vi "HFRR ADV v025 new software.vi"() -> ()   [LabVIEW 2025] (continued)
              n1908 = local write "Numeric 12"(w2274) -> ()
              n1909 = String Length(string=w2275) -> (length=w2277:i32)
              n1910 = Greater?(x=w2277, y=1) -> (0:w2273:bool)
            }
            n1911 = while {
              tunnel: w2248 -> [w2284]
              i -> [w2280]
              stop <- w2279 continue-if-true
              (unwired) TRUE ("line mode (F)")
              n1912 = Read from Text File "Read File"(file (use dialog)=w2284) -> (text=w2281:string)  [unwired: 3 in, 3 out]
              n1913 = local write "Numeric 13"(w2280) -> ()
              n1914 = String Length(string=w2281) -> (length=w2283:i32)
              n1915 = Greater?(x=w2283, y=1) -> (0:w2279:bool)
            }
            n1916 = String To Path(string=w2247) -> (path=w2255:path)
            n1917 = Open/Create/Replace File "Open File"(file path (use dialog)=w2255) -> (refnum out=w2251:refnum<file>)  [unwired: 5 in, 2 out]
            n1918 = while {
              tunnel: w2251 -> [w2266]
              i -> [w2262]
              stop <- w2261 continue-if-true
              (unwired) TRUE ("line mode (F)")
              n1919 = Read from Text File "Read File"(file (use dialog)=w2266) -> (text=w2263:string)  [unwired: 3 in, 3 out]
              n1920 = local write "Numeric 8"(w2262) -> ()
              n1921 = String Length(string=w2263) -> (length=w2265:i32)
              n1922 = Greater?(x=w2265, y=1) -> (0:w2261:bool)
            }
          }
          frame #1 {
            w2436 = FALSE ("ACTUAL   MERGE")
            # "Sample Temp"
            # "ECR"
            # "COF"
            # "Time\nCOF\nFF\nTemp"
            n1923 = case shown="True" w2309 {
              tunnel: [w2456 w2457] -> w2310
              frame False {
                n1924 = local read "string1"() -> (w2456:string)
              }
              frame True {
                n1925 = local read "String Indicator 4"() -> (w2457:string)
              }
            }
            n1926 = local read "string1 3"() -> (w2354:string)
            n1927 = String To Path(string=w2310) -> (path=w2441:path)
            n1928 = String To Path(string=w2354) -> (path=w2452:path)
            n1929 = local read "Numeric 12"() -> (w2438:i32)
            n1930 = local read "Numeric 8"() -> (w2440:i32)
            n1931 = local read "string1 2"() -> (w2355:string)
            n1932 = local read "string1 4"() -> (w2353:string)
            n1933 = Open/Create/Replace File "Open File"(file path (use dialog)=w2441) -> (refnum out=w2455:refnum<file>, error out=w2454:errorcluster)  [unwired: 5 in, 1 out]
            n1934 = Open/Create/Replace File "Open File"(file path (use dialog)=w2452) -> (refnum out=w2448:refnum<file>, error out=w2449:errorcluster)  [unwired: 5 in, 1 out]
            n1935 = for {
              N: w2440 -> [_]
              tunnel: w2455 -> [w2603]
              tunnel: w2454 -> [w2602]
              tunnel: [w2592] -> w2367 mode=indexing
              tunnel: [w2590] -> w2424 mode=indexing
              tunnel: [w2591] -> w2419 mode=indexing
              tunnel: w2436 -> [_]
              tunnel: [w2584] -> w2421 mode=indexing
              tunnel: [w2580] -> w2390 mode=indexing
              tunnel: [w2576] -> w2365 mode=indexing
              tunnel: [w2572] -> w2346 mode=indexing
              tunnel: [w2567] -> w2306 mode=indexing
              (unwired) TRUE ("line mode (F)")
              # "freq"
              # "Stroke"
              # "Time"
              # "CoF"
              # "Humidity"
              # "Temp"
              # "Air Temp"
              # "ECR"
              n1936 = Read from Text File "Read File"(file (use dialog)=w2603, error in=w2602) -> (text=w2568:string)  [unwired: 2 in, 3 out]
              n1937 = local write "String 6"(w2568) -> ()
              n1938 = String Subset(string=w2568, offset (0)=0, length (rest)=14 ("length (rest)")) -> (substring=w2596:string)
              n1939 = String Subset(string=w2568, offset (0)=35, length (rest)=9 ("length (rest)")) -> (substring=w2593:string)
              n1940 = String Subset(string=w2568, offset (0)=15, length (rest)=9 ("length (rest)")) -> (substring=w2599:string)
              n1941 = Fract/Exp String To Number(string=w2596) -> (number=w2592:dbl)  [unwired: 3 in, 1 out]
              n1942 = Fract/Exp String To Number(string=w2593) -> (number=w2591:dbl)  [unwired: 3 in, 1 out]
              n1943 = Fract/Exp String To Number(string=w2599) -> (number=w2590:dbl)  [unwired: 3 in, 1 out]
              n1944 = String Subset(string=w2568, offset (0)=85, length (rest)=9 ("length (rest)")) -> (substring=w2569:string)
              n1945 = String Subset(string=w2568, offset (0)=25, length (rest)=9 ("length (rest)")) -> (substring=w2575:string)
              n1946 = String Subset(string=w2568, offset (0)=55, length (rest)=9 ("length (rest)")) -> (substring=w2577:string)
              n1947 = String Subset(string=w2568, offset (0)=45, length (rest)=9 ("length (rest)")) -> (substring=w2583:string)
              n1948 = String Subset(string=w2568, offset (0)=65, length (rest)=9 ("length (rest)")) -> (substring=w2589:string)
              n1949 = Fract/Exp String To Number(string=w2575) -> (number=w2572:dbl)  [unwired: 3 in, 1 out]
              n1950 = Fract/Exp String To Number(string=w2569) -> (number=w2567:dbl)  [unwired: 3 in, 1 out]
              n1951 = Fract/Exp String To Number(string=w2577) -> (number=w2576:dbl)  [unwired: 3 in, 1 out]
              n1952 = Fract/Exp String To Number(string=w2583) -> (number=w2580:dbl)  [unwired: 3 in, 1 out]
              n1953 = Fract/Exp String To Number(string=w2589) -> (number=w2586:dbl)  [unwired: 3 in, 1 out]
              n1954 = Add(x=w2586, y=0.0) -> (x+y=w2584:dbl)
            }
            n1955 = for {
              N: w2438 -> [_]
              tunnel: w2449 -> [w2529]
              tunnel: w2448 -> [w2528]
              tunnel: [w2518] -> w2407 mode=indexing
              tunnel: [w2516] -> w2405 mode=indexing
              tunnel: [w2517] -> w2401 mode=indexing
              tunnel: w2436 -> [_]
              tunnel: [w2510] -> w2403 mode=indexing
              tunnel: [w2506] -> w2385 mode=indexing
              tunnel: [w2502] -> w2361 mode=indexing
              tunnel: [w2499] -> w2342 mode=indexing
              tunnel: [w2495] -> w2301 mode=indexing
              (unwired) 9 ("length (rest)")
              (unwired) 9 ("length (rest)")
              (unwired) TRUE ("line mode (F)")
              n1956 = Read from Text File "Read File"(file (use dialog)=w2528, error in=w2529) -> (text=w2496:string)  [unwired: 2 in, 3 out]
              n1957 = local write "String 8"(w2496) -> ()
              n1958 = String Subset(string=w2496, offset (0)=85) -> (substring=w2498:string)  [unwired: 1 in]
              n1959 = String Subset(string=w2496, offset (0)=35, length (rest)=9 ("length (rest)")) -> (substring=w2519:string)
              n1960 = String Subset(string=w2496, offset (0)=55, length (rest)=9 ("length (rest)")) -> (substring=w2504:string)
              n1961 = String Subset(string=w2496, offset (0)=25) -> (substring=w2500:string)  [unwired: 1 in]
              n1962 = String Subset(string=w2496, offset (0)=15, length (rest)=9 ("length (rest)")) -> (substring=w2525:string)
              n1963 = String Subset(string=w2496, offset (0)=0, length (rest)=14 ("length (rest)")) -> (substring=w2522:string)
              n1964 = String Subset(string=w2496, offset (0)=45, length (rest)=9 ("length (rest)")) -> (substring=w2509:string)
              n1965 = String Subset(string=w2496, offset (0)=65, length (rest)=9 ("length (rest)")) -> (substring=w2515:string)
              n1966 = Fract/Exp String To Number(string=w2498) -> (number=w2495:dbl)  [unwired: 3 in, 1 out]
              n1967 = Fract/Exp String To Number(string=w2519) -> (number=w2517:dbl)  [unwired: 3 in, 1 out]
              n1968 = Fract/Exp String To Number(string=w2504) -> (number=w2502:dbl)  [unwired: 3 in, 1 out]
              n1969 = Fract/Exp String To Number(string=w2500) -> (number=w2499:dbl)  [unwired: 3 in, 1 out]
              n1970 = Fract/Exp String To Number(string=w2525) -> (number=w2516:dbl)  [unwired: 3 in, 1 out]
              n1971 = Fract/Exp String To Number(string=w2522) -> (number=w2518:dbl)  [unwired: 3 in, 1 out]
              n1972 = Fract/Exp String To Number(string=w2509) -> (number=w2506:dbl)  [unwired: 3 in, 1 out]
              n1973 = Fract/Exp String To Number(string=w2515) -> (number=w2512:dbl)  [unwired: 3 in, 1 out]
              n1974 = Add(x=w2512, y=0.0) -> (x+y=w2510:dbl)
            }
            n1975 = String To Path(string=w2355) -> (path=w2453:path)
            n1976 = String To Path(string=w2353) -> (path=w2447:path)
            n1977 = local read "Numeric 11"() -> (w2437:i32)
            n1978 = local read "Numeric 13"() -> (w2439:i32)
            n1979 = Open/Create/Replace File "Open File"(file path (use dialog)=w2453) -> (refnum out=w2451:refnum<file>, error out=w2450:errorcluster)  [unwired: 5 in, 1 out]
            n1980 = Open/Create/Replace File "Open File"(file path (use dialog)=w2447) -> (refnum out=w2446:refnum<file>, error out=w2445:errorcluster)  [unwired: 5 in, 1 out]
            n1981 = for {
              N: w2437 -> [_]
              tunnel: w2451 -> [w2566]
              tunnel: w2450 -> [w2565]
              tunnel: [w2555] -> w2417 mode=indexing
              tunnel: [w2553] -> w2415 mode=indexing
              tunnel: [w2554] -> w2410 mode=indexing
              tunnel: w2436 -> [_]
              tunnel: [w2547] -> w2412 mode=indexing
              tunnel: [w2543] -> w2388 mode=indexing
              tunnel: [w2539] -> w2363 mode=indexing
              tunnel: [w2535] -> w2344 mode=indexing
              tunnel: [w2530] -> w2302 mode=indexing
              (unwired) TRUE ("line mode (F)")
              n1982 = Read from Text File "Read File"(file (use dialog)=w2566, error in=w2565) -> (text=w2531:string)  [unwired: 2 in, 3 out]
              n1983 = local write "String 7"(w2531) -> ()
              n1984 = String Subset(string=w2531, offset (0)=85, length (rest)=9 ("length (rest)")) -> (substring=w2534:string)
              n1985 = String Subset(string=w2531, offset (0)=35, length (rest)=9 ("length (rest)")) -> (substring=w2556:string)
              n1986 = String Subset(string=w2531, offset (0)=55, length (rest)=9 ("length (rest)")) -> (substring=w2542:string)
              n1987 = String Subset(string=w2531, offset (0)=25, length (rest)=9 ("length (rest)")) -> (substring=w2536:string)
              n1988 = String Subset(string=w2531, offset (0)=45, length (rest)=9 ("length (rest)")) -> (substring=w2544:string)
              n1989 = String Subset(string=w2531, offset (0)=0, length (rest)=14 ("length (rest)")) -> (substring=w2559:string)
              n1990 = String Subset(string=w2531, offset (0)=15, length (rest)=9 ("length (rest)")) -> (substring=w2562:string)
              n1991 = String Subset(string=w2531, offset (0)=65, length (rest)=9 ("length (rest)")) -> (substring=w2548:string)
              n1992 = Fract/Exp String To Number(string=w2534) -> (number=w2530:dbl)  [unwired: 3 in, 1 out]
              n1993 = Fract/Exp String To Number(string=w2556) -> (number=w2554:dbl)  [unwired: 3 in, 1 out]
              n1994 = Fract/Exp String To Number(string=w2542) -> (number=w2539:dbl)  [unwired: 3 in, 1 out]
              n1995 = Fract/Exp String To Number(string=w2536) -> (number=w2535:dbl)  [unwired: 3 in, 1 out]
              n1996 = Fract/Exp String To Number(string=w2544) -> (number=w2543:dbl)  [unwired: 3 in, 1 out]
              n1997 = Fract/Exp String To Number(string=w2559) -> (number=w2555:dbl)  [unwired: 3 in, 1 out]
              n1998 = Fract/Exp String To Number(string=w2562) -> (number=w2553:dbl)  [unwired: 3 in, 1 out]
              n1999 = Fract/Exp String To Number(string=w2548) -> (number=w2551:dbl)  [unwired: 3 in, 1 out]
              n2000 = Add(x=w2551, y=0.0) -> (x+y=w2547:dbl)
            }
            n2001 = for {
              N: w2439 -> [_]
              tunnel: w2446 -> [w2494]
              tunnel: w2445 -> [w2493]
              tunnel: [w2483] -> w2399 mode=indexing
              tunnel: [w2482] -> w2392 mode=indexing
              tunnel: w2436 -> [_]
              tunnel: [w2471] -> w2397 mode=indexing
              tunnel: [w2476] -> w2394 mode=indexing
              tunnel: [w2472] -> w2384 mode=indexing
              tunnel: [w2467] -> w2359 mode=indexing
              tunnel: [w2463] -> w2340 mode=indexing
              tunnel: [w2458] -> w2300 mode=indexing
              (unwired) 1.0 ("x")
              (unwired) TRUE ("line mode (F)")
              n2002 = Read from Text File "Read File"(file (use dialog)=w2494, error in=w2493) -> (text=w2459:string)  [unwired: 2 in, 3 out]
              n2003 = local write "String 12"(w2459) -> ()
              n2004 = String Subset(string=w2459, offset (0)=85, length (rest)=9 ("length (rest)")) -> (substring=w2461:string)
              n2005 = String Subset(string=w2459, offset (0)=35, length (rest)=9 ("length (rest)")) -> (substring=w2484:string)
              n2006 = String Subset(string=w2459, offset (0)=55, length (rest)=9 ("length (rest)")) -> (substring=w2469:string)
              n2007 = String Subset(string=w2459, offset (0)=25, length (rest)=9 ("length (rest)")) -> (substring=w2465:string)
              n2008 = String Subset(string=w2459, offset (0)=45, length (rest)=9 ("length (rest)")) -> (substring=w2474:string)
              n2009 = String Subset(string=w2459, offset (0)=15, length (rest)=9 ("length (rest)")) -> (substring=w2490:string)
              n2010 = String Subset(string=w2459, offset (0)=0, length (rest)=14 ("length (rest)")) -> (substring=w2487:string)
              n2011 = String Subset(string=w2459, offset (0)=65, length (rest)=9 ("length (rest)")) -> (substring=w2477:string)
              n2012 = Fract/Exp String To Number(string=w2461) -> (number=w2458:dbl)  [unwired: 3 in, 1 out]
              n2013 = Fract/Exp String To Number(string=w2484) -> (number=w2482:dbl)  [unwired: 3 in, 1 out]
              n2014 = Fract/Exp String To Number(string=w2469) -> (number=w2467:dbl)  [unwired: 3 in, 1 out]
              n2015 = Fract/Exp String To Number(string=w2465) -> (number=w2463:dbl)  [unwired: 3 in, 1 out]
              n2016 = Fract/Exp String To Number(string=w2474) -> (number=w2472:dbl)  [unwired: 3 in, 1 out]
              n2017 = Fract/Exp String To Number(string=w2490) -> (number=w2471:dbl)  [unwired: 3 in, 1 out]
              n2018 = Fract/Exp String To Number(string=w2487) -> (number=w2483:dbl)  [unwired: 3 in, 1 out]
              n2019 = Fract/Exp String To Number(string=w2477) -> (number=w2480:dbl)  [unwired: 3 in, 1 out]
              n2020 = Add(x=w2480, y=0.0) -> (x+y=w2476:dbl)
            }
            n2021 = Delete From Array(array=w2342, index=0) -> (array with subset deleted=w2315:dbl[])  [unwired: 1 in, 1 out]
            n2022 = Delete From Array(array=w2405, index=0) -> (array with subset deleted=w2378:dbl[])  [unwired: 1 in, 1 out]
            n2023 = Delete From Array(array=w2385, index=0) -> (array with subset deleted=w2373:dbl[])  [unwired: 1 in, 1 out]
            n2024 = Delete From Array(array=w2403, index=0) -> (array with subset deleted=w2404:dbl[])  [unwired: 1 in, 1 out]
            n2025 = call-poly <vilib>:"Mean.vi"("X"=w2315) -> ("mean"=→"КОФ2 4":dbl)  [unwired: 1 out]
            n2026 = call-poly <vilib>:"Mean.vi"("X"=w2378) -> ("mean"=→"КОФ3":dbl)  [unwired: 1 out]
            n2027 = call-poly <vilib>:"Mean.vi"("X"=w2373) -> ("mean"=→"CP3":dbl)  [unwired: 1 out]
            n2028 = Delete From Array(array=w2367, index=0) -> (array with subset deleted=w2294:dbl[])  [unwired: 1 in, 1 out]
            n2029 = Delete From Array(array=w2306, index=0) -> (array with subset deleted=w2293:dbl[])  [unwired: 1 in, 1 out]
            n2030 = Delete From Array(array=w2346, index=0) -> (array with subset deleted=w2317:dbl[])  [unwired: 1 in, 1 out]
            n2031 = Delete From Array(array=w2424, index=0) -> (array with subset deleted=w2379:dbl[])  [unwired: 1 in, 1 out]
            n2032 = Delete From Array(array=w2390, index=0) -> (array with subset deleted=w2375:dbl[])  [unwired: 1 in, 1 out]
            "array w/ subset deleted" <- w2375
            n2033 = Delete From Array(array=w2421, index=0) -> (array with subset deleted=w2422:dbl[])  [unwired: 1 in, 1 out]
            n2034 = call-poly <vilib>:"Mean.vi"("X"=w2317) -> ("mean"=→"КОФ2 2":dbl)  [unwired: 1 out]
            n2035 = call-poly <vilib>:"Mean.vi"("X"=w2379) -> ("mean"=→"КОФ1":dbl)  [unwired: 1 out]
            n2036 = Bundle "Bundle"(w2294, w2293) -> (w2299:cluster{dbl[], dbl[]})  [unwired: 1 in]
            n2037 = Bundle "Bundle"(w2294, w2422) -> (w2286:cluster{dbl[], dbl[]})  [unwired: 1 in]
            n2038 = Delete From Array(array=w2301, index=0) -> (array with subset deleted=w2289:dbl[])  [unwired: 1 in, 1 out]
            n2039 = Delete From Array(array=w2302, index=0) -> (array with subset deleted=w2291:dbl[])  [unwired: 1 in, 1 out]
            n2040 = Delete From Array(array=w2412, index=0) -> (array with subset deleted=w2413:dbl[])  [unwired: 1 in, 1 out]
            n2041 = Delete From Array(array=w2300, index=0) -> (array with subset deleted=w2287:dbl[])  [unwired: 1 in, 1 out]
            n2042 = Delete From Array(array=w2394, index=0) -> (array with subset deleted=w2395:dbl[])  [unwired: 1 in, 1 out]
            n2043 = Delete From Array(array=w2419, index=0) -> (array with subset deleted=w2325:dbl[])  [unwired: 1 in, 1 out]
            n2044 = Delete From Array(array=w2365, index=0) -> (array with subset deleted=w2321:dbl[])  [unwired: 1 in, 1 out]
            n2045 = Delete From Array(array=w2401, index=0) -> (array with subset deleted=w2323:dbl[])  [unwired: 1 in, 1 out]
            n2046 = Delete From Array(array=w2361, index=0) -> (array with subset deleted=w2319:dbl[])  [unwired: 1 in, 1 out]
            n2047 = Delete From Array(array=w2410, index=0) -> (array with subset deleted=w2324:dbl[])  [unwired: 1 in, 1 out]
            n2048 = Delete From Array(array=w2363, index=0) -> (array with subset deleted=w2320:dbl[])  [unwired: 1 in, 1 out]
            n2049 = Delete From Array(array=w2344, index=0) -> (array with subset deleted=w2316:dbl[])  [unwired: 1 in, 1 out]
            n2050 = Delete From Array(array=w2388, index=0) -> (array with subset deleted=w2374:dbl[])  [unwired: 1 in, 1 out]
            n2051 = Delete From Array(array=w2415, index=0) -> (array with subset deleted=w2376:dbl[])  [unwired: 1 in, 1 out]
            n2052 = Delete From Array(array=w2392, index=0) -> (array with subset deleted=w2322:dbl[])  [unwired: 1 in, 1 out]
            n2053 = Delete From Array(array=w2359, index=0) -> (array with subset deleted=w2318:dbl[])  [unwired: 1 in, 1 out]
            n2054 = Delete From Array(array=w2340, index=0) -> (array with subset deleted=w2314:dbl[])  [unwired: 1 in, 1 out]
            n2055 = Delete From Array(array=w2384, index=0) -> (array with subset deleted=w2372:dbl[])  [unwired: 1 in, 1 out]
            n2056 = Delete From Array(array=w2397, index=0) -> (array with subset deleted=w2377:dbl[])  [unwired: 1 in, 1 out]
            n2057 = Delete From Array(array=w2407, index=0) -> (array with subset deleted=w2290:dbl[])  [unwired: 1 in, 1 out]
            n2058 = Delete From Array(array=w2417, index=0) -> (array with subset deleted=w2292:dbl[])  [unwired: 1 in, 1 out]
            n2059 = Delete From Array(array=w2399, index=0) -> (array with subset deleted=w2288:dbl[])  [unwired: 1 in, 1 out]
            n2060 = Bundle "Bundle"(w2294, w2325) -> (w2312:cluster{dbl[], dbl[]})  [unwired: 1 in]
            n2061 = Bundle "Bundle"(w2294, w2379) -> (w2313:cluster{dbl[], dbl[]})  [unwired: 1 in]
            n2062 = Bundle "Bundle"(w2325, w2321) -> (w2327:cluster{dbl[], dbl[]})  [unwired: 1 in]
            n2063 = Bundle "Bundle"(w2290, w2289) -> (w2297:cluster{dbl[], dbl[]})  [unwired: 1 in]
            n2064 = Bundle "Bundle"(w2323, w2319) -> (w2329:cluster{dbl[], dbl[]})  [unwired: 1 in]
            n2065 = Bundle "Bundle"(w2290, w2323) -> (w2433:cluster{dbl[], dbl[]})  [unwired: 1 in]
            n2066 = Bundle "Bundle"(w2290, w2319) -> (w2357:cluster{dbl[], dbl[]})  [unwired: 1 in]
            n2067 = Bundle "Bundle"(w2290, w2378) -> (w2443:cluster{dbl[], dbl[]})  [unwired: 1 in]
            n2068 = Bundle "Bundle"(w2290, w2373) -> (w2381:cluster{dbl[], dbl[]})  [unwired: 1 in]
            n2069 = Bundle "Bundle"(w2290, w2404) -> (w2428:cluster{dbl[], dbl[]})  [unwired: 1 in]
            n2070 = Bundle "Bundle"(w2324, w2320) -> (w2328:cluster{dbl[], dbl[]})  [unwired: 1 in]
            n2071 = Bundle "Bundle"(w2292, w2291) -> (w2298:cluster{dbl[], dbl[]})  [unwired: 1 in]
            n2072 = Bundle "Bundle"(w2292, w2324) -> (w2435:cluster{dbl[], dbl[]})  [unwired: 1 in]
            n2073 = Bundle "Bundle"(w2292, w2320) -> (w2358:cluster{dbl[], dbl[]})  [unwired: 1 in]
            n2074 = Bundle "Bundle"(w2292, w2374) -> (w2382:cluster{dbl[], dbl[]})  [unwired: 1 in]
            n2075 = Bundle "Bundle"(w2292, w2376) -> (w2444:cluster{dbl[], dbl[]})  [unwired: 1 in]
            n2076 = Bundle "Bundle"(w2292, w2413) -> (w2426:cluster{dbl[], dbl[]})  [unwired: 1 in]
            n2077 = Bundle "Bundle"(w2322, w2318) -> (w2330:cluster{dbl[], dbl[]})  [unwired: 1 in]
            n2078 = Bundle "Bundle"(w2288, w2287) -> (w2296:cluster{dbl[], dbl[]})  [unwired: 1 in]
            n2079 = Bundle "Bundle"(w2288, w2322) -> (w2434:cluster{dbl[], dbl[]})  [unwired: 1 in]
            n2080 = Bundle "Bundle"(w2288, w2318) -> (w2356:cluster{dbl[], dbl[]})  [unwired: 1 in]
            n2081 = Bundle "Bundle"(w2288, w2372) -> (w2380:cluster{dbl[], dbl[]})  [unwired: 1 in]
            n2082 = Bundle "Bundle"(w2288, w2377) -> (w2442:cluster{dbl[], dbl[]})  [unwired: 1 in]
            n2083 = Bundle "Bundle"(w2288, w2395) -> (w2427:cluster{dbl[], dbl[]})  [unwired: 1 in]
            n2084 = call-poly <vilib>:"Mean.vi"("X"=w2375) -> ("mean"=→"CP1":dbl)  [unwired: 1 out]
            n2085 = call-poly <vilib>:"Mean.vi"("X"=w2316) -> ("mean"=→"КОФ2 3":dbl)  [unwired: 1 out]
            n2086 = call-poly <vilib>:"Mean.vi"("X"=w2374) -> ("mean"=→"CP2":dbl)  [unwired: 1 out]
            n2087 = call-poly <vilib>:"Mean.vi"("X"=w2376) -> ("mean"=→"КОФ2":dbl)  [unwired: 1 out]
            n2088 = call-poly <vilib>:"Mean.vi"("X"=w2314) -> ("mean"=→"КОФ2 5":dbl)  [unwired: 1 out]
            n2089 = call-poly <vilib>:"Mean.vi"("X"=w2372) -> ("mean"=→"CP4":dbl)  [unwired: 1 out]
            n2090 = call-poly <vilib>:"Mean.vi"("X"=w2377) -> ("mean"=→"КОФ4":dbl)  [unwired: 1 out]
            n2091 = Bundle "Bundle"(w2294, w2321) -> (w2285:cluster{dbl[], dbl[]})  [unwired: 1 in]
            n2092 = Bundle "Bundle"(w2294, w2375) -> (w2308:cluster{dbl[], dbl[]})  [unwired: 1 in]
            n2093 = Build Array "Build Array"(w2285, w2308) -> (w2311:cluster{dbl[], dbl[]}[])
            "XY Graph 17" <- w2311
            n2094 = Build Array "Build Array"(w2299, w2298, w2297, w2296) -> (→"Frequency ( Hz )":cluster{dbl[], dbl[]}[])
            n2095 = Build Array "Build Array"(w2327, w2328, w2329, w2330) -> (→"Air Temp ( °C ) vs Humidity ( % RH )":cluster{dbl[], dbl[]}[])
            n2096 = Build Array "Build Array"(w2312, w2435, w2433, w2434) -> (→"Air Temperature  ( °C )":cluster{dbl[], dbl[]}[])
            n2097 = Build Array "Build Array"(w2285, w2358, w2357, w2356) -> (→"Humidity ( %RH )":cluster{dbl[], dbl[]}[])
            n2098 = Build Array "Build Array"(w2313, w2444, w2443, w2442) -> (→"Coefficient Of Friction":cluster{dbl[], dbl[]}[])
            n2099 = Build Array "Build Array"(w2308, w2382, w2381, w2380) -> (→"Sample Temperature ( °C )":cluster{dbl[], dbl[]}[])
            n2100 = Build Array "Build Array"(w2286, w2426, w2428, w2427) -> (→"XY Graph 13":cluster{dbl[], dbl[]}[])
            n2101 = Bundle "Bundle"(w2294, w2317) -> (w2339:cluster{dbl[], dbl[]})  [unwired: 1 in]
            n2102 = Bundle "Bundle"(w2290, w2315) -> (w2337:cluster{dbl[], dbl[]})  [unwired: 1 in]
            n2103 = Bundle "Bundle"(w2292, w2316) -> (w2338:cluster{dbl[], dbl[]})  [unwired: 1 in]
            n2104 = Bundle "Bundle"(w2288, w2314) -> (w2336:cluster{dbl[], dbl[]})  [unwired: 1 in]
            n2105 = Build Array "Build Array"(w2339, w2338, w2337, w2336) -> (→"Stroke ( mm )":cluster{dbl[], dbl[]}[])
            n2106 = local write "XY Graph 16"(w2311) -> ()
          }
          frame #2 {
          }
          frame #3 {
            n2107 = local write "Numeric 8"(0 ("Numeric 8")) -> ()
            n2108 = local write "Numeric 11"(0 ("Numeric 11")) -> ()
            n2109 = local write "Numeric 12"(0 ("Numeric 12")) -> ()
            n2110 = local write "Numeric 13"(0 ("Numeric 13")) -> ()
            n2111 = property on="OPEN" class="Bool (strict)"("Visible"=TRUE) -> ()  [unwired: 2 in, 2 out]
            n2112 = local read "String Control 2"() -> (w2611:string)
            n2113 = local read "String Control 4"() -> (w2610:string)
            n2114 = local read "String Control 6"() -> (w2609:string)
            n2115 = local read "String Control 8"() -> (w2608:string)
            n2116 = Match Pattern(string=w2611, regular expression="Samples / cycle :- ") -> (after substring=w2625:string)  [unwired: 1 in, 3 out]
            n2117 = Match Pattern(string=w2611, regular expression="Frequency :- ") -> (after substring=w2644:string)  [unwired: 1 in, 3 out]
            n2118 = Match Pattern(string=w2610, regular expression="Samples / cycle :- ") -> (after substring=w2621:string)  [unwired: 1 in, 3 out]
            n2119 = Match Pattern(string=w2610, regular expression="Frequency :- ") -> (after substring=w2639:string)  [unwired: 1 in, 3 out]
            n2120 = Match Pattern(string=w2609, regular expression="Samples / cycle :- ") -> (after substring=w2617:string)  [unwired: 1 in, 3 out]
            n2121 = Match Pattern(string=w2609, regular expression="Frequency :- ") -> (after substring=w2634:string)  [unwired: 1 in, 3 out]
            n2122 = Match Pattern(string=w2608, regular expression="Samples / cycle :- ") -> (after substring=w2613:string)  [unwired: 1 in, 3 out]
            n2123 = Match Pattern(string=w2608, regular expression="Frequency :- ") -> (after substring=w2629:string)  [unwired: 1 in, 3 out]
            n2124 = String Subset(string=w2625, length (rest)=6 ("length (rest)")) -> (substring=w2627:string)  [unwired: 1 in]
            n2125 = String Subset(string=w2644, length (rest)=9 ("length (rest)")) -> (substring=w2646:string)  [unwired: 1 in]
            n2126 = String Subset(string=w2621, length (rest)=6 ("length (rest)")) -> (substring=w2623:string)  [unwired: 1 in]
            n2127 = String Subset(string=w2639, length (rest)=9 ("length (rest)")) -> (substring=w2641:string)  [unwired: 1 in]
            n2128 = String Subset(string=w2617, length (rest)=6 ("length (rest)")) -> (substring=w2619:string)  [unwired: 1 in]
            n2129 = String Subset(string=w2634, length (rest)=9 ("length (rest)")) -> (substring=w2636:string)  [unwired: 1 in]
            n2130 = String Subset(string=w2613, length (rest)=6 ("length (rest)")) -> (substring=w2615:string)  [unwired: 1 in]
            n2131 = String Subset(string=w2629, length (rest)=9 ("length (rest)")) -> (substring=w2631:string)  [unwired: 1 in]
            n2132 = Fract/Exp String To Number(string=w2627) -> (number=w2607:dbl)  [unwired: 3 in, 1 out]
            n2133 = Fract/Exp String To Number(string=w2646) -> (number=w2647:dbl)  [unwired: 3 in, 1 out]
            n2134 = Fract/Exp String To Number(string=w2623) -> (number=w2606:dbl)  [unwired: 3 in, 1 out]
            n2135 = Fract/Exp String To Number(string=w2641) -> (number=w2642:dbl)  [unwired: 3 in, 1 out]
            n2136 = Fract/Exp String To Number(string=w2619) -> (number=w2605:dbl)  [unwired: 3 in, 1 out]
            n2137 = Fract/Exp String To Number(string=w2636) -> (number=w2637:dbl)  [unwired: 3 in, 1 out]
            n2138 = Fract/Exp String To Number(string=w2615) -> (number=w2604:dbl)  [unwired: 3 in, 1 out]
            n2139 = Fract/Exp String To Number(string=w2631) -> (number=w2632:dbl)  [unwired: 3 in, 1 out]
            n2140 = local write "sample1"(w2607) -> ()
            n2141 = local write "freq1"(w2647) -> ()
            n2142 = local write "sample2"(w2606) -> ()
            n2143 = local write "freq2"(w2642) -> ()
            n2144 = local write "sample3"(w2605) -> ()
            n2145 = local write "freq3"(w2637) -> ()
            n2146 = local write "sample4"(w2604) -> ()
            n2147 = local write "freq 4"(w2632) -> ()
          }
        }
      }
    }
    n2148 = case shown="True" w2096 {
      selector: w2096 -> [_ w2224]
      frame False {
      }
      frame True {
        n2149 = Not(x=w2224) -> (.not. x?=w2220:bool)
        n2150 = local write "service 3"(w2220) -> ()
        n2151 = local write "OPEN 6"(w2220) -> ()
        n2152 = call <vilib>:"System Exec.vi"("wait until completion? (T)"=TRUE, "command line"="C:\\LAB-IQ\\Scar View.exe") -> ("error out"=→"error out 5":errorcluster)  [unwired: 6 in, 3 out]
      }
    }
    n2153 = case shown="\"About\"" w2107 {
      frame "Acquire", Default {
        w2960 = 0.2 ("y")
        w2965 = 1.0 ("y")
        w2966 = 0.8 ("y")
        # "Elapsed time\ncof\nstroke\nAir temp\nTemp\nHumidity"
        n2154 = disable-structure shown="Disabled" {
          frame Disabled {
            n2155 = local read "Flag"() -> (w2983:dbl)
            n2156 = local read "RUN"() -> (w2980:bool)
            n2157 = Not(x=w2980) -> (.not. x?=w2979:bool)
            n2158 = Equal?(x=w2983, y=10.0) -> (x = y?=w2981:bool)
            n2159 = And(x=w2981, y=w2979) -> (x .and. y?=w2978:bool)
            n2160 = case shown="True" w2978 {
              frame False {
              }
              frame True {
                w2984 = FALSE ("Heater Button")
                n2161 = local write "Humidity"(w2984) -> ()
                n2162 = local write "Heater Button"(w2984) -> ()
              }
            }
          }
          frame Enabled {
          }
        }
        n2163 = disable-structure shown="Disabled" {
          frame Disabled {
            n2164 = case shown="True" {
              selector: _ -> [_ _]
              frame False {
              }
              frame True {
                w3075 = TRUE ("Heater")
                n2165 = local write "Humidity"(w3075) -> ()
                n2166 = local write "Heater Button"(w3075) -> ()
                n2167 = local read "TEST STANDARD"() -> (w3078:T3)
                n2168 = local read "TEST STANDARD"() -> (w3073:T3)
                n2169 = Equal?(x=w3078, y=enum16{"ASTM D6079", "ISO 12156", "Custom"}."ISO 12156" ("Test Standard")) -> (x = y?=w3076:bool)
                n2170 = Equal?(x=w3073, y=enum16{"ASTM D6079", "ISO 12156", "Custom"}."ASTM D6079" ("Test Standard")) -> (x = y?=w3072:bool)
                n2171 = case shown="True" w3076 {
                  frame False {
                  }
                  frame True {
                    n2172 = local write "Heater"(TRUE ("Heater")) -> ()
                    n2173 = local write "airtempflg"(FALSE ("airtempflg")) -> ()
                  }
                }
                n2174 = case shown="True" w3072 {
                  frame False {
                  }
                  frame True {
                    n2175 = local write "Heater"(FALSE ("Heater")) -> ()
                    n2176 = local write "airtempflg"(TRUE ("airtempflg")) -> ()
                  }
                }
              }
            }
          }
          frame Enabled {
          }
        }
        n2177 = stacked-sequence {
          frame #0 {
            n2178 = case shown="True" "RST FF" {
              frame False {
              }
              frame True {
                w3141 = 0.0 ("X Scale.Range:Maximum")
                n2179 = property on="Frictional Force ( N )" class="WFChart (strict)"("XScale.Maximum"=600.0 ("X Scale.Range:Maximum"), "XScale.Minimum"=w3141, "YScale.Maximum"=10.0 ("Y Scale.Range:Maximum"), "YScale.Minimum"=w3141) -> ()  [unwired: 2 in, 2 out]
              }
            }
          }
          frame #1 {
            n2180 = case shown="True" "RST TEMP" {
              frame False {
              }
              frame True {
                n2181 = property on="Temperature ( Deg C )" class="WFChart (strict)"("XScale.Minimum"=0.0 ("X Scale.Range:Minimum"), "XScale.Maximum"=600.0 ("X Scale.Range:Maximum"), "YScale.Minimum"=0.0 ("Y Scale.Range:Minimum"), "YScale.Maximum"=100.0 ("Y Scale.Range:Maximum")) -> ()  [unwired: 2 in, 2 out]
              }
            }
          }
          frame #2 {
            n2182 = case shown="True" "RSTCOF" {
              frame False {
              }
              frame True {
                n2183 = property on="Coefficient of Friction" class="WFChart (strict)"("XScale.Minimum"=0.0 ("X Scale.Range:Minimum"), "XScale.Maximum"=600.0 ("X Scale.Range:Maximum"), "YScale.Maximum"=1.0 ("X Scale.Range:Minimum"), "YScale.Minimum"=0.0 ("X Scale.Range:Minimum")) -> ()  [unwired: 2 in, 2 out]
              }
            }
          }
          frame #3 {
            n2184 = case shown="True" "RSTCOF 2" {
              frame False {
              }
              frame True {
                (unwired) 100.0 ("Y Scale.Range:Maximum")
                (unwired) 0.0 ("Y Scale.Range:Minimum")
                (unwired) 600.0 ("X Scale.Range:Maximum")
                (unwired) 0.0 ("X Scale.Range:Minimum")
              }
            }
          }
          frame #4 {
            n2185 = case shown="True" "RSTCOF 3" {
              frame False {
              }
              frame True {
                n2186 = property on="Electrical Contact Resistance ( % )" class="WFChart (strict)"("XScale.Minimum"=0.0 ("X Scale.Range:Minimum"), "XScale.Maximum"=600.0 ("X Scale.Range:Maximum"), "YScale.Minimum"=0.0 ("Y Scale.Range:Minimum"), "YScale.Maximum"=100.0 ("Y Scale.Range:Maximum")) -> ()  [unwired: 2 in, 2 out]
              }
            }
          }
        }
        n2187 = disable-structure shown="Disabled" {
          frame Disabled {
            n2188 = case shown="True" {
              selector: _ -> [_ _]
              frame False {
              }
              frame True {
                n2189 = local read "zflag 2"() -> (w3042:dbl)
                n2190 = local read "yflag"() -> (w3044:dbl)
                n2191 = Equal?(x=w3044, y=2.0 ("tflag")) -> (x = y?=w3046:bool)
                n2192 = Equal?(x=w3042, y=3.0 ("tflag")) -> (x = y?=w3045:bool)
                n2193 = And(x=w3046, y=w3045) -> (x .and. y?=w3040:bool)
                n2194 = case shown="True" w3040 {
                  frame False {
                  }
                  frame True {
                    w3071 = 0.0 ("zflag")
                    n2195 = local write "zflag"(w3071) -> ()
                    n2196 = local write "zflag 2"(w3071) -> ()
                    n2197 = Delete(path (use dialog)=path "C:/LAB-IQ-NXT/WO 2449 TT.sig" ("file path (dialog if empty)")) -> (deleted path=w3070:path)  [unwired: 4 in, 2 out]
                    n2198 = Delete(path (use dialog)=path "C:/LAB-IQ-NXT/WO 2449 TRH.sig" ("file path (dialog if empty)")) -> (deleted path=w3065:path)  [unwired: 4 in, 2 out]
                    n2199 = local read "SEN.RUN HRS"() -> (w3057:dbl)
                    n2200 = local read "SENSOR TIME"() -> (w3055:dbl)
                    n2201 = call <vilib>:"compatOverwrite.vi"("overwrite (F)"=TRUE) -> ("overwrite?"=w3047:T28)
                    n2202 = call <vilib>:"compatOverwrite.vi"("overwrite (F)"=TRUE) -> ("overwrite?"=w3051:T28)
                    n2203 = local read "Total No. of Tests"() -> (w3058:dbl)
                    n2204 = Add(x=w3055, y=w3057) -> (x+y=w3056:dbl)
                    "SEN.RUN HRS" <- w3056
                    n2205 = Open/Create/Replace File(file path (use dialog)=w3070, operation (0:open)=w3047) -> (refnum out=w3048:refnum<file>, error out=w3049:errorcluster)  [unwired: 4 in, 1 out]
                    n2206 = Open/Create/Replace File(file path (use dialog)=w3065, operation (0:open)=w3051) -> (refnum out=w3052:refnum<file>, error out=w3053:errorcluster)  [unwired: 4 in, 1 out]
                    n2207 = Deny Access(4:w3049, 6:T26."deny none" ("deny mode (2)"), 7:w3048) -> (3:w3069:refnum<file>)  [unwired: 1 out]
                    n2208 = Deny Access(4:w3053, 6:T26."deny none" ("deny mode (2)"), 7:w3052) -> (3:w3061:refnum<file>)  [unwired: 1 out]
                    n2209 = Number To Decimal String(number=w3058) -> (decimal integer string=w3066:string)  [unwired: 1 in]
                    n2210 = Number To Decimal String(number=w3056) -> (decimal integer string=w3062:string)  [unwired: 1 in]
                    n2211 = Write to Binary File(file (use dialog)=w3069, data=w3066, 5:FALSE ("prepend array or string size? (T)")) -> ()  [unwired: 3 in, 3 out]
                    n2212 = Write to Binary File(file (use dialog)=w3061, data=w3062, 5:FALSE ("prepend array or string size? (T)")) -> ()  [unwired: 3 in, 3 out]
                  }
                }
              }
            }
          }
          frame Enabled {
          }
        }
        n2213 = local read "RUN"() -> (w2969:bool)
        n2214 = local read "run replace"() -> (w2973:bool)
        n2215 = local read "run replace"() -> (w2972:bool)
        n2216 = case shown="True" w2969 {
          frame False {
            n2217 = local write "run replace"(FALSE ("run replace")) -> ()
          }
          frame True {
            "run replace" <- TRUE ("run replace")
          }
        }
        n2218 = local read "RUN"() -> (w2977:bool)
        n2219 = local read "Set Temp"() -> (w2939:dbl)
        n2220 = local read "SetTemp"() -> (w2941:dbl)
        n2221 = case shown="False" w2977 {
          tunnel: [FALSE ("TEST RUNNING") TRUE ("TEST RUNNING")] -> w2976
          frame False {
            w3160 = 0.0 ("Flag")
            n2222 = local write "Elapsed time"(0.0 ("elapsedtime")) -> ()
            n2223 = local write "Time Remaining"(w3160) -> ()
            n2224 = local write "Flag"(w3160) -> ()
            n2225 = local write "Remaining Time"(w3160) -> ()
          }
          frame True {
            n2226 = local write "Flag"(10.0 ("Flag")) -> ()
          }
        }
        n2227 = case shown="False" w2973 {
          frame False {
            n2228 = local read "zflag"() -> (→"zflag 2":dbl)
            n2229 = local write "yflag"(2.0 ("tflag")) -> ()
            n2230 = local write "FLAG 4"(0.0 ("FLAG")) -> ()
          }
          frame True {
            n2231 = local write "yflag"(1.0 ("tflag")) -> ()
            n2232 = local write "zflag"(3.0 ("zflag")) -> ()
          }
        }
        n2233 = local read "acq 2"() -> (w2971:bool)
        n2234 = local read "AIR TEMP"() -> (w2934:dbl)
        n2235 = local read "Amb temp"() -> (w2938:dbl)
        n2236 = case shown="True" "Save & Continue" {
          frame False {
          }
          frame True {
            "acq 2" <- TRUE ("acq 2")
          }
        }
        n2237 = local read "Set Rh"() -> (w2940:dbl)
        n2238 = Add(x=w2941, y=w2966) -> (x+y=w2967:dbl)
        n2239 = Subtract(x=w2941, y=w2966) -> (x-y=w2968:dbl)
        n2240 = Add(x=w2939, y=w2960) -> (x+y=w2961:dbl)
        n2241 = Subtract(x=w2939, y=w2960) -> (x-y=w2962:dbl)
        n2242 = And(x=w2971, y=w2972) -> (x .and. y?=w2970:bool)
        n2243 = Greater Or Equal?(x=w2934, y=15.0) -> (x >= y?=w2935:bool)
        "powstat" <- w2935
        n2244 = local read "Humidity ( %RH )"() -> (w2937:dbl)
        n2245 = case shown="True" "Save & Continue" {
          frame False {
          }
          frame True {
            n2246 = while {
              tunnel: "0123456789abcdefghijklmnopqrstuvwxyzABCDEFGHIJKLMNOPQRSTUVWXYZ" ("string 2") -> [w3131]
              shift-right: [w3129] -> w3124
              shift-left: "" -> [w3128]
              i -> [w3138]
              stop <- w3137 stop-if-true
              n2247 = Random Number (0-1)() -> (number: 0 to 1=w3132:dbl)
              n2248 = Multiply(x=w3132, y=62.0) -> (x*y=w3134:dbl)
              n2249 = Decrement(x="Length") -> (x-1=w3127:i16)
              n2250 = To Word Integer(number=w3134) -> (16bit integer=w3135:i16)
              n2251 = String Subset(string=w3131, offset (0)=w3135, length (rest)=1 ("length (rest)")) -> (substring=w3130:string)
              n2252 = Greater Or Equal?(x=w3138, y=w3127) -> (x >= y?=w3137:bool)
              n2253 = Concatenate Strings(w3130, w3128) -> (w3129:string)
            }
            n2254 = local write "UUID"(w3124) -> ()
          }
        }
        n2255 = In Range and Coerce(upper limit=w2967, x=w2938, lower limit=w2968) -> (In Range?=w2957:bool)  [unwired: 1 out]
        n2256 = Add(x=w2940, y=w2965) -> (x+y=w2964:dbl)
        n2257 = Subtract(x=w2940, y=w2965) -> (x-y=w2963:dbl)
        n2258 = local read "TEMP"() -> (w2936:dbl)
        n2259 = case shown="True" "Save & Continue" {
          frame False {
          }
          frame True {
            n2260 = local read "Operator ID"() -> (w3455:string)
            n2261 = local read "FILE"() -> (w3461:string)
            n2262 = String Length(string=w3461) -> (length=w3459:i32)
            n2263 = String Length(string=w3455) -> (length=w3456:i32)
            n2264 = Greater?(x=w3459, y=0) -> (0:w3458:bool)
            n2265 = Greater?(x=w3456, y=0) -> (0:w3454:bool)
            n2266 = And(x=w3458, y=w3454) -> (x .and. y?=w3453:bool)
            n2267 = case shown="True" w3453 {
              frame False {
                n2268 = stacked-sequence {
                  frame #0 {
                    n2269 = One Button Dialog(message="Please Enter a File Name and Operator ID to save data !", button name ("OK")="Ok") -> ()  [unwired: 1 out]
                  }
                  frame #1 {
                    n2270 = local write "Save & Continue"(FALSE ("OK Button")) -> ()
                  }
                }
                n2271 = local write "Save & Continue"(FALSE ("OK Button")) -> ()
              }
              frame True {
                n2272 = stacked-sequence {
                  frame #0 {
                    n2273 = local read "FILE"() -> (w3467:string)
                    n2274 = call "file check.vi"("file name in"=w3467) -> ("file name out"=w3466:string)  [unwired: 9 in, 1 out]
                    n2275 = call <vilib>:"Application Directory.vi"() -> ("Application Directory"=w3477:path)
                    n2276 = Build Path(base path=w3477, name or relative path="data") -> (appended path=w3476:path)
                    n2277 = call <vilib>:"Trim Whitespace.vi"("string"=w3466) -> ("trimmed string"=w3474:string)  [unwired: 1 in]
                    n2278 = call <vilib>:"Trim Whitespace.vi"("string"=w3466) -> ("trimmed string"=w3475:string)  [unwired: 1 in]
                    n2279 = List Folder(path=w3476) -> (folder names=w3472:string[])  [unwired: 3 in, 3 out]
                    n2280 = Match Pattern(string=w3474, regular expression="_(") -> (before substring=w3471:string)  [unwired: 1 in, 3 out]
                    n2281 = for {
                      tunnel: w3472 -> [w3486] mode=indexing
                      tunnel: w3471 -> [w3484]
                      shift-right: [w3482] -> w3469
                      shift-left: bool[] [] -> [w3483]
                      n2282 = Match Pattern(string=w3486, regular expression="_(") -> (before substring=w3485:string)  [unwired: 1 in, 3 out]
                      n2283 = Equal?(x=w3485, y=w3484) -> (x = y?=w3481:bool)
                      n2284 = case shown="True" w3481 {
                        tunnel: w3481 -> [_ w3489]
                        tunnel: w3483 -> [w3488 w3491]
                        tunnel: [w3488 w3490] -> w3482
                        frame False {
                        }
                        frame True {
                          n2285 = Insert Into Array(array=w3491, new element=w3489) -> (w3490:bool[])  [unwired: 1 in]
                        }
                      }
                    }
                    n2286 = Equal?(x=w3472, y=w3471) -> (x = y?=w3480:bool[])
                    n2287 = Or Array Elements(Boolean array=w3480) -> (logical OR=w3479:bool)
                    n2288 = Array Size(array=w3469) -> (size(s)=w3468:i32)
                    n2289 = case shown="True" w3479 {
                      tunnel: w3475 -> [_ w3499]
                      tunnel: w3468 -> [_ w3492]
                      frame False {
                      }
                      frame True {
                        n2290 = Number To Decimal String(number=w3492) -> (decimal integer string=w3495:string)  [unwired: 1 in]
                        n2291 = Search/Split String(string=w3499, search string/char (-)="_(" ("regular expression")) -> (substring before match=w3497:string)  [unwired: 1 in, 2 out]
                        n2292 = Concatenate Strings(w3497, "_(" ("regular expression"), w3495, ")" ("regular expression")) -> (w3493:string)
                        n2293 = local write "FILE"(w3493) -> ()
                      }
                    }
                  }
                  frame #1 {
                    w3501 = 0.0
                    w3514 = cluster{"y":dbl, dbl, "y":dbl}[] [] ("History Data")
                    w3515 = FALSE ("Heater Button")
                    (unwired) ")!" ("string")
                    (unwired) ")" ("string")
                    w3513 = dbl[] [] ("History Data")
                    w3519 = "\r"
                    # "C:\\WinDucom\\Data\\"
                    # "C:\\LAB-IQ-NXT\\data"
                    n2294 = local write "Humidity ( %RH )"(w3501) -> ()
                    n2295 = local write "Frequency ( Hz )"(w3501) -> ()
                    n2296 = local write "Stroke 3"(w3501) -> ()
                    n2297 = local write "speedop"(0.0 ("PIDclk 2")) -> ()
                    n2298 = local write "Set Temp 2"(65.0 ("Set Temp 2")) -> ()
                    n2299 = local write "AIR TEMP"(w3501) -> ()
                    n2300 = local write "clk"(0.0 ("clk")) -> ()
                    n2301 = local write "Stroke 4"(w3501) -> ()
                    n2302 = local write "COF 2"(w3501) -> ()
                    n2303 = local write "TEMP"(w3501) -> ()
                    n2304 = local write "ecr 3"(w3501) -> ()
                    n2305 = local write "FF 3"(w3501) -> ()
                    n2306 = local write "FF 2"(w3501) -> ()
                    n2307 = property on="Humidity ( %RH )" class="WFChart (strict)"("History Data"=w3513) -> ()  [unwired: 2 in, 2 out]
                    n2308 = property on="Coefficient of Friction" class="WFChart (strict)"("History Data"=w3513) -> ()  [unwired: 2 in, 2 out]
                    n2309 = property on="Coefficient of Friction" class="WFChart (strict)"("History Data"=w3513) -> ()  [unwired: 2 in, 2 out]
                    n2310 = property on="Frictional Force ( N )" class="WFChart (strict)"("History Data"=w3513) -> ()  [unwired: 2 in, 2 out]
                    n2311 = property on="Electrical Contact Resistance ( % )" class="WFChart (strict)"("History Data"=w3513) -> ()  [unwired: 2 in, 2 out]
                    n2312 = property on="Electrical Contact Resistance ( % )" class="WFChart (strict)"("History Data"=w3513) -> ()  [unwired: 2 in, 2 out]
                    n2313 = property on="Temperature ( Deg C )" class="WFChart (strict)"("History Data"=w3513) -> ()  [unwired: 2 in, 2 out]
                    n2314 = property on="Frictional Force ( N )" class="WFChart (strict)"("History Data"=w3513) -> ()  [unwired: 2 in, 2 out]
                    n2315 = property on="Coefficient of Friction" class="WFChart (strict)"("History Data"=w3513) -> ()  [unwired: 2 in, 2 out]
                    n2316 = property on="Frictional Force ( N )" class="WFChart (strict)"("History Data"=w3513) -> ()  [unwired: 2 in, 2 out]
                    n2317 = property on="Electrical Contact Resistance ( % )" class="WFChart (strict)"("History Data"=w3513) -> ()  [unwired: 2 in, 2 out]
                    n2318 = property on="Temperature ( Deg C )" class="WFChart (strict)"("History Data"=w3513) -> ()  [unwired: 2 in, 2 out]
                    n2319 = property on="Humidity ( %RH )" class="WFChart (strict)"("History Data"=w3513) -> ()  [unwired: 2 in, 2 out]
                    n2320 = property on="Stroke ( mm )" class="WFChart (strict)"("History Data"=w3514) -> ()  [unwired: 2 in, 2 out]
                    n2321 = property on="Stroke ( mm )" class="WFChart (strict)"("History Data"=w3514) -> ()  [unwired: 2 in, 2 out]
                    n2322 = local write "Humidity"(w3515) -> ()
                    n2323 = local write "Heater Button"(w3515) -> ()
                    n2324 = local read "FILE"() -> (w3509:string)
                    n2325 = disable-structure shown="Enabled" {
                      disable-tunnel: [w3554 _] -> w3500
                      frame Enabled {
                        n2326 = local read "NORMAL LOAD"() -> (w3554:dbl)
                      }
                      frame Disabled {
                      }
                    }
                    n2327 = call "file check.vi"("file name in"=w3509) -> ("error out"=w3512:errorcluster, "file name out"=w3506:string)  [unwired: 9 in]
                    n2328 = call "FILE PATH CREATION.vi"("error in"=w3512, "FILE NAME :"=w3506) -> ("FILE OUT"=w3505:path)  [unwired: 8 in, 1 out]
                    n2329 = Concatenate Strings(w3506, ".dgf" ("Substring")) -> (w3511:string)
                    n2330 = Concatenate Strings(w3506, ".duf" ("Substring")) -> (w3507:string)
                    n2331 = Multiply(x=w3500, y=1.0) -> (x*y=w3533:dbl)
                    n2332 = Build Path(base path=w3505, name or relative path=w3511) -> (appended path=w3504:path)
                    n2333 = Build Path(base path=w3505, name or relative path=w3507) -> (appended path=w3503:path)
                    n2334 = Number To Fractional String(number=w3533, width (-)=i16 5, precision (6)=i16 2) -> (F-format string=w3541:string)  [unwired: 1 in]
                    n2335 = local read "Fuel Discription :"() -> (w3529:string)
                    n2336 = local read "Batch Ref Num :"() -> (w3517:string)
                    n2337 = Get Date/Time String(date format (0)=enum16{"short", "long", "abbreviated"}."short") -> (date string=w3552:string, time string=w3549:string)  [unwired: 2 in]
                    n2338 = local read "Remarks :"() -> (w3528:string)
                    n2339 = Concatenate Strings("Load :- " ("Substring"), w3541, " grams ," ("Substring")) -> (w3540:string)
                    n2340 = local read "String 41"() -> (w3520:string)
                    n2341 = Concatenate Strings(w3529) -> (w3530:string)
                    n2342 = Concatenate Strings(w3517) -> (w3516:string)
                    n2343 = Concatenate Strings("tested by") -> (w3524:string)
                    n2344 = Concatenate Strings("(" ("Substring"), w3552, ")" ("Substring"), w3549) -> (w3522:string)
                    "concatenated string" <- w3522
                    n2345 = Concatenate Strings(w3528, "," ("string")) -> (w3527:string)
                    n2346 = Concatenate Strings("  TIME;      COF;       STROKE;     AIR TEMP;  TEMP;  HUMIDITY;  ECR; PID-OUT; FREQUENCY" ("Substring"), "\r") -> (w3536:string)
                    n2347 = Concatenate Strings(w3520, w3519, "Fuel Discription :-" ("Substring"), w3530, w3519, w3540, w3519, "Batch Ref Num :-" ("Substring"), w3516, w3519, " Remarks :- " ("Substring"), w3527, w3519, " Date :- " ("Substring"), w3522, w3519, "Tested By :-" ("Substring"), w3524) -> (w3534:string)
                    "REMARKS" <- w3534
                    n2348 = call <vilib>:"Write Characters To File.vi"("append to file? (new file:F)"=FALSE, "character string"=w3536, "file path (dialog if empty)"=w3504) -> ()  [unwired: 2 in, 1 out]
                    n2349 = call <vilib>:"Write Characters To File.vi"("append to file? (new file:F)"=FALSE, "character string"=w3534, "file path (dialog if empty)"=w3503) -> ()  [unwired: 2 in, 1 out]
                  }
                  frame #2 {
                    n2350 = local write "Cycles elapsed"(0 ("Cycles elapsed")) -> ()
                    n2351 = local write "cyclecount"(0 ("cyclecount")) -> ()
                    n2352 = local write "Save & Continue"(FALSE ("OK")) -> ()
                    n2353 = local write "autostrtflg"(TRUE ("autostrtflg")) -> ()
                    n2354 = local write "Save"(FALSE ("Save")) -> ()
                    n2355 = Get Date/Time In Seconds() -> (seconds since 1Jan1904=w3559:timestamp)
                    n2356 = To Double Precision Float(number=w3559) -> (double precision float=w3558:dbl)
                    n2357 = local write "acq timer"(w3558) -> ()
                    n2358 = One Button Dialog(message="Please ensure sample is mounted properly and machine is ready in all aspects for testing !", button name ("OK")="Ok") -> ()  [unwired: 1 out]
                  }
                  frame #3 {
                    n2359 = stacked-sequence {
                      frame #0 {
                        n2360 = local write "Main Dashboard Buttons"(T1."Dashboard" ("Main Dashboard Buttons")) -> ()
                        n2361 = local write "Main Tab"(T2."Acquire" ("Main Tab")) -> ()
                      }
                      frame #1 {
                        n2362 = local write "EVENT LOG"("" ("EVENT LOG")) -> ()
                      }
                      frame #2 {
                        n2363 = Wait (ms)(milliseconds to wait=u32 50) -> ()  [unwired: 1 out]
                      }
                      frame #3 {
                        n2364 = disable-structure shown="Disabled" {
                          frame Disabled {
                            n2365 = local read "EVENT LOG"() -> (w3571:string)
                            n2366 = call "Event Log.vi"("Content"="Test Details", "EVENT LOG"=w3571) -> ("EVENT LOG"=w3570:string)  [unwired: 8 in, 1 out]
                            n2367 = local write "EVENT LOG"(w3570) -> ()
                          }
                          frame Enabled {
                          }
                        }
                      }
                      frame #4 {
                        n2368 = Wait (ms)(milliseconds to wait=u32 50) -> ()  [unwired: 1 out]
                      }
                      frame #5 {
                        n2369 = local read "FILE"() -> (w3573:string)
                        n2370 = Concatenate Strings("File Name :" ("Content"), w3573) -> (w3574:string)
                        n2371 = local read "EVENT LOG"() -> (w3577:string)
                        n2372 = call "Event Log.vi"("Content"=w3574, "EVENT LOG"=w3577) -> ("EVENT LOG"=w3576:string)  [unwired: 8 in, 1 out]
                        n2373 = local write "EVENT LOG"(w3576) -> ()
                      }
                      frame #6 {
                        n2374 = Wait (ms)(milliseconds to wait=u32 50) -> ()  [unwired: 1 out]
                      }
                      frame #7 {
                        n2375 = local read "Batch Ref Num :"() -> (w3579:string)
                        n2376 = Concatenate Strings("Batch Ref No :" ("Content"), w3579) -> (w3580:string)
                        n2377 = local read "EVENT LOG"() -> (w3583:string)
                        n2378 = call "Event Log.vi"("Content"=w3580, "EVENT LOG"=w3583) -> ("EVENT LOG"=w3582:string)  [unwired: 8 in, 1 out]
                        n2379 = local write "EVENT LOG"(w3582) -> ()
                      }
                      frame #8 {
                        n2380 = Wait (ms)(milliseconds to wait=u32 50) -> ()  [unwired: 1 out]
                      }
                      frame #9 {
                        n2381 = local read "tested by"() -> (w3585:string)
                        n2382 = Concatenate Strings("Tested By :" ("Content"), w3585) -> (w3586:string)
                        n2383 = local read "EVENT LOG"() -> (w3589:string)
                        n2384 = call "Event Log.vi"("Content"=w3586, "EVENT LOG"=w3589) -> ("EVENT LOG"=w3588:string)  [unwired: 8 in, 1 out]
                        n2385 = local write "EVENT LOG"(w3588) -> ()
                      }
                      frame #10 {
                        n2386 = Wait (ms)(milliseconds to wait=u32 50) -> ()  [unwired: 1 out]
                      }
                      frame #11 {
                        n2387 = local read "TEST STANDARD"() -> (w3592:T3)
                        n2388 = case shown="\"ASTM D6079\", Default" w3592 {
                          tunnel: ["ASTM D6079" "ISO 12156" "CEC F-096-A-06" "Custom"] -> w3591
                          frame "ASTM D6079", Default {
                          }
                          frame "ISO 12156" {
                          }
                          frame "CEC F-096-A-06" {
                          }
                          frame "Custom" {
                          }
                        }
                        n2389 = Concatenate Strings("Test Standard :" ("Content"), w3591) -> (w3593:string)
                        n2390 = local read "EVENT LOG"() -> (w3596:string)
                        n2391 = call "Event Log.vi"("Content"=w3593, "EVENT LOG"=w3596) -> ("EVENT LOG"=w3595:string)  [unwired: 8 in, 1 out]
                        n2392 = local write "EVENT LOG"(w3595) -> ()
                      }
                      frame #12 {
                        n2393 = Wait (ms)(milliseconds to wait=u32 50) -> ()  [unwired: 1 out]
                      }
                      frame #13 {
                        n2394 = local read "Fuel Discription :"() -> (w3602:string)
                        n2395 = Concatenate Strings("Fuel Description :" ("Content"), w3602) -> (w3603:string)
                        n2396 = local read "EVENT LOG"() -> (w3606:string)
                        n2397 = call "Event Log.vi"("Content"=w3603, "EVENT LOG"=w3606) -> ("EVENT LOG"=w3605:string)  [unwired: 8 in, 1 out]
                        n2398 = local write "EVENT LOG"(w3605) -> ()
                      }
                      frame #14 {
                        n2399 = Wait (ms)(milliseconds to wait=u32 50) -> ()  [unwired: 1 out]
                      }
                      frame #15 {
                        n2400 = local read "Remarks :"() -> (w3608:string)
                        n2401 = Concatenate Strings("Remarks :" ("Content"), w3608) -> (w3609:string)
                        n2402 = local read "EVENT LOG"() -> (w3612:string)
                        n2403 = call "Event Log.vi"("Content"=w3609, "EVENT LOG"=w3612) -> ("EVENT LOG"=w3611:string)  [unwired: 8 in, 1 out]
                        n2404 = local write "EVENT LOG"(w3611) -> ()
                      }
                      frame #16 {
                        n2405 = Wait (ms)(milliseconds to wait=u32 50) -> ()  [unwired: 1 out]
                      }
                      frame #17 {
                        n2406 = local read "Operator ID"() -> (w3614:string)
                        n2407 = Concatenate Strings("Operator ID :" ("Content"), w3614) -> (w3616:string)
                        n2408 = local read "EVENT LOG"() -> (w3618:string)
                        n2409 = call "Event Log.vi"("Content"=w3616, "EVENT LOG"=w3618) -> ("EVENT LOG"=w3617:string)  [unwired: 8 in, 1 out]
                        n2410 = local write "EVENT LOG"(w3617) -> ()
                      }
                      frame #18 {
                        n2411 = Wait (ms)(milliseconds to wait=u32 50) -> ()  [unwired: 1 out]
                      }
                      frame #19 {
                        n2412 = disable-structure shown="Disabled" {
                          frame Disabled {
                            n2413 = local read "EVENT LOG"() -> (w3622:string)
                            n2414 = call "Event Log.vi"("Content"="Test Parameter", "EVENT LOG"=w3622) -> ("EVENT LOG"=w3621:string)  [unwired: 8 in, 1 out]
                            n2415 = local write "EVENT LOG"(w3621) -> ()
                          }
                          frame Enabled {
                          }
                        }
                      }
                      frame #20 {
                        n2416 = Wait (ms)(milliseconds to wait=u32 50) -> ()  [unwired: 1 out]
                      }
                      frame #21 {
                        n2417 = local read "Set Hz"() -> (w3626:dbl)
                        n2418 = Number To Fractional String(number=w3626, precision (6)=i16 2) -> (F-format string=w3625:string)  [unwired: 2 in]
                        n2419 = Concatenate Strings("Set Frequency [Hz] :" ("Content"), w3625) -> (w3628:string)
                        n2420 = local read "EVENT LOG"() -> (w3630:string)
                        n2421 = call "Event Log.vi"("Content"=w3628, "EVENT LOG"=w3630) -> ("EVENT LOG"=w3629:string)  [unwired: 8 in, 1 out]
                        n2422 = local write "EVENT LOG"(w3629) -> ()
                      }
                      frame #22 {
                        n2423 = Wait (ms)(milliseconds to wait=u32 50) -> ()  [unwired: 1 out]
                      }
                      frame #23 {
                        n2424 = local read "NORMAL LOAD"() -> (w3633:dbl)
                        n2425 = Number To Fractional String(number=w3633, precision (6)=i16 2) -> (F-format string=w3634:string)  [unwired: 2 in]
                        n2426 = Concatenate Strings("Applied Load [grams] :" ("Content"), w3634) -> (w3636:string)
                        n2427 = local read "EVENT LOG"() -> (w3638:string)
                        n2428 = call "Event Log.vi"("Content"=w3636, "EVENT LOG"=w3638) -> ("EVENT LOG"=w3637:string)  [unwired: 8 in, 1 out]
                        n2429 = local write "EVENT LOG"(w3637) -> ()
                      }
                      frame #24 {
                        n2430 = Wait (ms)(milliseconds to wait=u32 50) -> ()  [unwired: 1 out]
                      }
                      frame #25 {
                        n2431 = local read "Set Strk"() -> (w3641:dbl)
